vi "Enqueue Local Message.vi"(7 "Priority (F)":bool, 8 "error in":errorcluster, 9 "Data":variant, 10 "Message":string, 11 "Msg queue in":refnum<queue>) -> (0 "error out":errorcluster, 3 "queue out":refnum<queue>)   [LabVIEW 2021, in "Architecture.lvlib"]
doc: "This VI queues a message to a local message queue. Used to enqueue states in a single module state machine."
uses:
  Architecture.lvlib
  Typedefs/Message.ctl
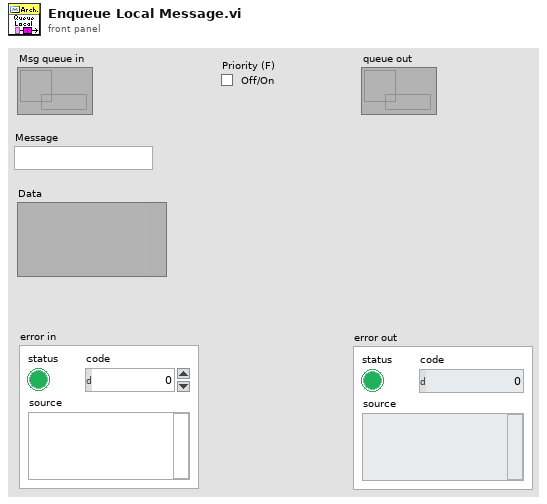
[diagram p1: front panel]
types:
  T1 = typedef "Architecture.lvlib/Message.ctl" = cluster{"Message":string, "Data":variant, "syn":bool}
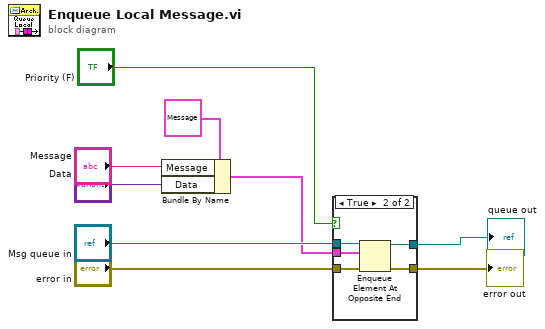
[diagram p0: block diagram]
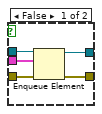
[diagram p2: hidden frame]
diagram:
  n1 = Bundle By Name(cluster=T1 {"Message"="", "Data"=variant, "syn"=FALSE} ("element"), "Message"="Message", "Data"="Data") -> (w4:T1)
  n2 = case shown="True" "Priority (F)" {
    tunnel: "Msg queue in" -> [w14 w17]
    tunnel: "error in" -> [w13 w19]
    tunnel: [w12 w18] -> w6
    tunnel: [w11 w16] -> w5
    tunnel: w4 -> [w10 w15]
    frame False {
      n3 = Enqueue Element(queue=w14, element=w10, error in (no error)=w13) -> (queue out=w11:refnum<queue>, error out=w12:errorcluster)  [unwired: 1 in, 1 out]
    }
    frame True {
      n4 = Enqueue Element At Opposite End(queue=w17, element=w15, error in (no error)=w19) -> (queue out=w16:refnum<queue>, error out=w18:errorcluster)  [unwired: 1 in, 1 out]
    }
  }
  "error out" <- w6
  "queue out" <- w5
